vi "Status TimerList (Start).vi"(8 "error in (no error)":errorcluster, 10 "Address (0)":i32, 11 "VISA resource name":refnum<visa-resource-name>) -> (0 "error out":errorcluster, 2 "Start Timer":T1 {"Start-Date (s)" format="%<%Y/%m/%d>T"; "Start-Time (s)" format="%<%H:%M>t"}, 3 "VISA resource name out":refnum<visa-resource-name>)   [LabVIEW 2016, in "Environment Chamber.lvlib" / "Climatic Chamber.lvlib"]
doc: "<b>Timer content monitor</b>\n\nReturns the settings of the Start Timer."
uses:
  Climatic Chamber.lvlib
  Private/Type Defs/Start_End Timer Cluster.ctl
  Private/Type Defs/Start Mode Enum.ctl
  Private/Type Defs/Operation_Stop Mode Enum.ctl
  Private/Type Defs/TimerNumber Enum.ctl
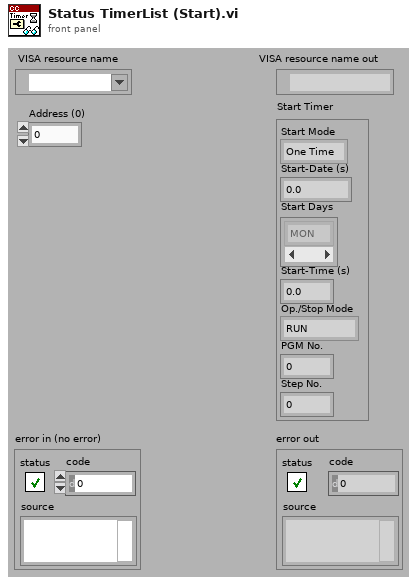
[diagram p1: front panel]
types:
  T1 = typedef "Environment Chamber.lvlib/Climatic Chamber.lvlib/Start_End Timer Cluster.ctl" = cluster{"Start Mode":T2, "Start-Date (s)":dbl, "Start Days":enum16{"MON", "TUE", "WED", "THU", "FRI", "SAT", "SUN"}[], "Start-Time (s)":dbl, "Op./Stop Mode":T3, "PGM No.":i32, "Step No.":i32}
  T2 = typedef "Environment Chamber.lvlib/Climatic Chamber.lvlib/Start Mode Enum.ctl" = enum16{"One Time", "Weekly", "Daily"}
  T3 = typedef "Environment Chamber.lvlib/Climatic Chamber.lvlib/Operation_Stop Mode Enum.ctl" = enum16{"RUN", "CONSTANT", "STANDBY", "OFF"}
  T4 = typedef "Environment Chamber.lvlib/Climatic Chamber.lvlib/TimerNumber Enum.ctl" = enum16{"Quick Timer", "Start Timer", "End Timer"}
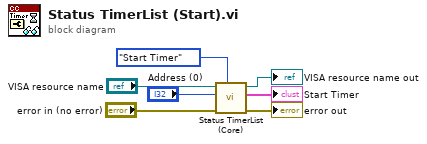
[diagram p0: block diagram]
diagram:
  n1 = call "Status TimerList (Core).vi"("Timer Number"=TimerNumber_Enum."Start Timer", "error in (no error)"="error in (no error)", "Address (0)"="Address (0)", "VISA resource name"="VISA resource name") -> ("error out"=→"error out":errorcluster, "Start Timer"=→"Start Timer":T1, "VISA resource name out"=→"VISA resource name out":refnum<visa-resource-name>)  [unwired: 3 in, 2 out]
